vi "Spartan HTTP Load Global Server Configuration.vi"(8 "error in (no error)":errorcluster, 11 "lvhttp.conf":path=path "") -> (0 "error out":errorcluster)   [LabVIEW 2011]
uses:
  ITK EXT/http/http0.llb/HTTP LVHTTP Global.vi
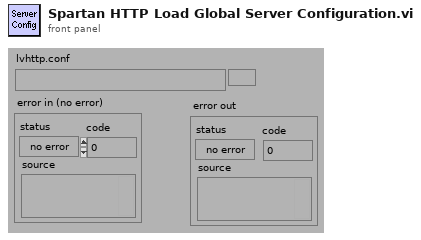
[diagram p1: front panel]
types:
  T1 = typedef "Keyed Array.ctl" = cluster{"keys":string[], "values":string[]}
  T2 = cluster{"[0]":path, "[1]":path, "[2]":path, "[3]":path, "[4]":path, "[5]":path, "[6]":path}
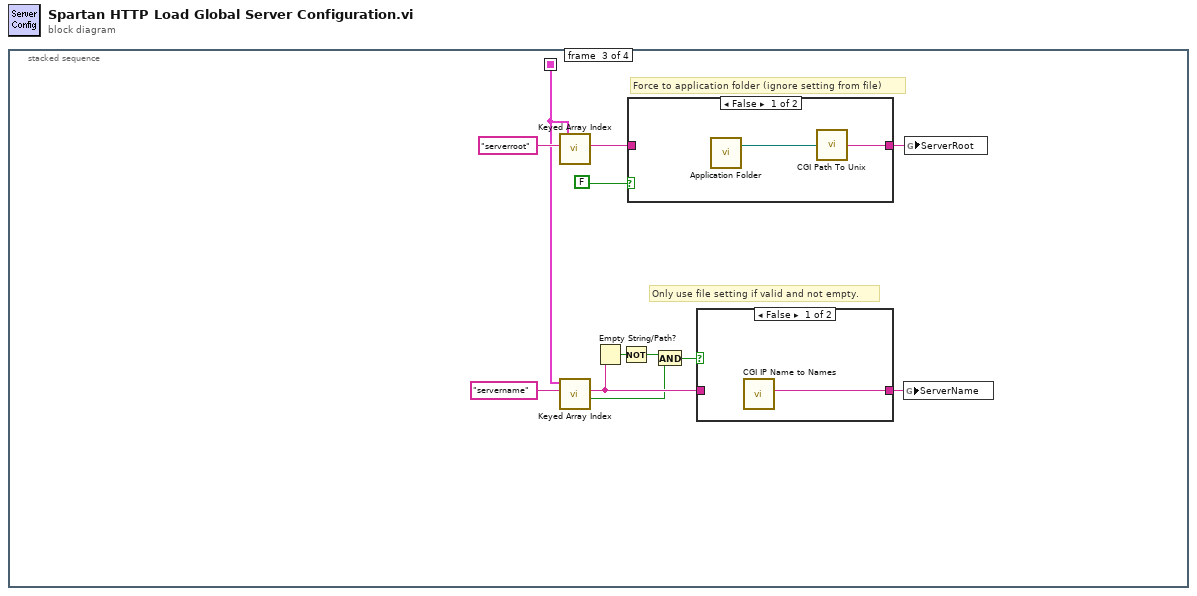
[diagram p0: block diagram]
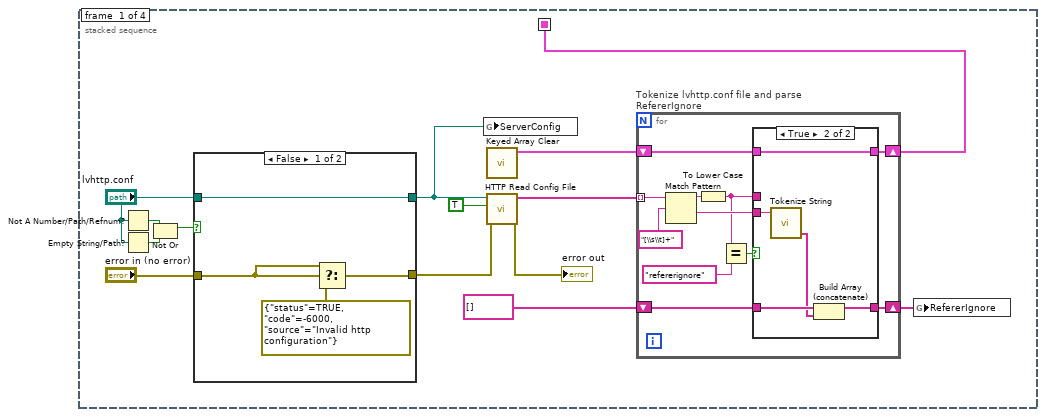
[diagram p2: hidden frame]
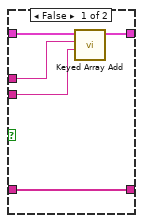
[diagram p4: hidden frame]
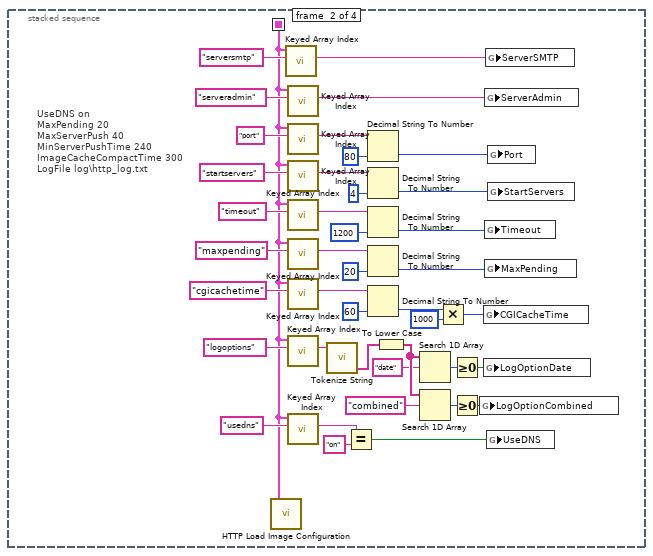
[diagram p5: hidden frame]
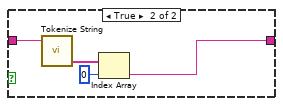
[diagram p7: hidden frame]
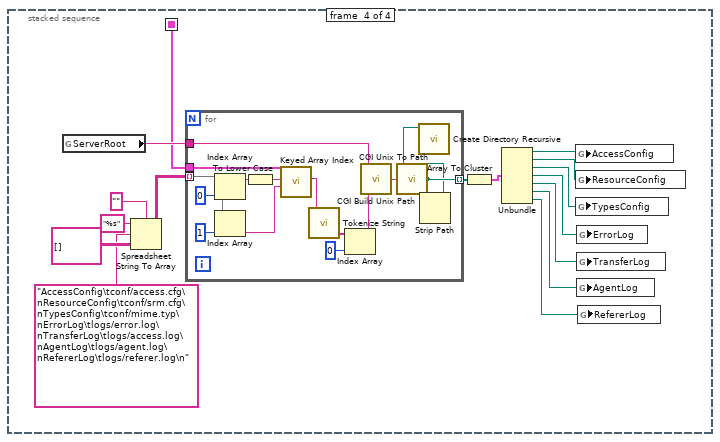
[diagram p8: hidden frame]
diagram:
  n1 = stacked-sequence {
    seq-local: [w9 _ _ _] -> [_ w42 w90 w104]
    frame #0 {
      n2 = Not A Number/Path/Refnum?(number/path/refnum="lvhttp.conf") -> (NaN/Path/Refnum?=w3:bool)
      n3 = Empty String/Path?(string/path="lvhttp.conf") -> (empty?=w4:bool)
      n4 = Not Or(1:w4, 2:w3) -> (0:w1:bool)
      n5 = case shown="False" w1 {
        tunnel: [w15 w20] -> w6
        tunnel: "lvhttp.conf" -> [w15 w20]
        tunnel: "error in (no error)" -> [w18 w19]
        tunnel: [w16 w19] -> w5
        frame False {
          n6 = Select(t=w18, s=w18, f=errorcluster {"status"=TRUE, "code"=-6000, "source"="Invalid http configuration"} ("error out")) -> (s? t:f=w16:errorcluster)
        }
        frame True {
        }
      }
      n7 = global write "HTTP LVHTTP Global.vi" "ServerConfig"(w6) -> ()
      n8 = call "Keyed Array Clear.vi"() -> ("array out"=w10:T1)  [unwired: 1 in, 6 out]
      n9 = call "HTTP Read Config File.vi"("error in (no error)"=w5, "skip blank lines (F)"=TRUE, "config file path"=w6) -> ("error out"=→"error out":errorcluster, "lines"=w13:string[])  [unwired: 7 out]
      n10 = for "Tokenize lvhttp.conf file and parse RefererIgnore" {
        shift-right: [w28] -> w9
        shift-left: w10 -> [w29]
        tunnel: w13 -> [w25] mode=indexing
        shift-right: [w26] -> w11
        shift-left: string[] [] -> [w27]
        n11 = Match Pattern(string=w25, regular expression="[\\s\\t]+") -> (before substring=w24:string, after substring=w23:string)  [unwired: 3 out]
        n12 = To Lower Case(string=w24) -> (all lower case string=w21:string)
        n13 = Equal?(x=w21, y="refererignore") -> (x = y?=w30:bool)
        n14 = case shown="True" w30 {
          tunnel: w29 -> [w36 w41]
          tunnel: w21 -> [w35 _]
          tunnel: [w33 w41] -> w28
          tunnel: w27 -> [w34 w40]
          tunnel: [w34 w39] -> w26
          tunnel: w23 -> [w32 w38]
          frame False {
            n15 = call "Keyed Array Add.vi"("value"=w32, "key"=w35, "array in"=w36) -> ("array out"=w33:T1)  [unwired: 1 in, 3 out]
          }
          frame True {
            n16 = call "Tokenize String.vi"("input string"=w38) -> ("token array"=w37:string[])  [unwired: 1 in, 3 out]
            n17 = Build Array (concatenate)(w40, w37) -> (w39:string[])
          }
        }
      }
      n18 = global write "HTTP LVHTTP Global.vi" "RefererIgnore"(w11) -> ()
    }
    frame #1 {
      # "UseDNS\ton\nMaxPending\t20\nMaxServerPush\t40\nMinServerPushTime 240\nImageCacheCompactTime\t300\nLogFile\tlog\\http_log.txt"
      n19 = call "HTTP Load Image Configuration.vi"("array in"=w42) -> ()  [unwired: 7 out]
      n20 = call "Keyed Array Index.vi"("key"="serversmtp", "array in"=w42) -> ("value"=w44:string)  [unwired: 2 in, 3 out]
      n21 = call "Keyed Array Index.vi"("key"="serveradmin", "array in"=w42) -> ("value"=w73:string)  [unwired: 2 in, 3 out]
      n22 = call "Keyed Array Index.vi"("key"="port", "array in"=w42) -> ("value"=w78:string)  [unwired: 2 in, 3 out]
      n23 = call "Keyed Array Index.vi"("key"="startservers", "array in"=w42) -> ("value"=w76:string)  [unwired: 2 in, 3 out]
      n24 = call "Keyed Array Index.vi"("key"="timeout", "array in"=w42) -> ("value"=w77:string)  [unwired: 2 in, 3 out]
      n25 = call "Keyed Array Index.vi"("key"="maxpending", "array in"=w42) -> ("value"=w67:string)  [unwired: 2 in, 3 out]
      n26 = call "Keyed Array Index.vi"("key"="cgicachetime", "array in"=w42) -> ("value"=w50:string)  [unwired: 2 in, 3 out]
      n27 = call "Keyed Array Index.vi"("key"="logoptions", "array in"=w42) -> ("value"=w60:string)  [unwired: 2 in, 3 out]
      n28 = call "Keyed Array Index.vi"("key"="usedns", "array in"=w42) -> ("value"=w64:string)  [unwired: 2 in, 3 out]
      n29 = call "Tokenize String.vi"("input string"=w60) -> ("token array"=w59:string[])  [unwired: 1 in, 3 out]
      n30 = Equal?(x=w64, y="on") -> (x = y?=w62:bool)
      n31 = Decimal String To Number(string=w78, default (0L)=u16 80) -> (number=w70:u16)  [unwired: 2 out]
      n32 = Decimal String To Number(string=w76, default (0L)=4) -> (number=w71:i32)  [unwired: 2 out]
      n33 = Decimal String To Number(string=w77, default (0L)=1200) -> (number=w72:i32)  [unwired: 2 out]
      n34 = Decimal String To Number(string=w67, default (0L)=20) -> (number=w69:i32)  [unwired: 2 out]
      n35 = Decimal String To Number(string=w50, default (0L)=60) -> (number=w48:i32)  [unwired: 2 out]
      n36 = To Lower Case(string=w59) -> (all lower case string=w58:string[])
      n37 = Search 1D Array(1D array=w58, element="date") -> (index of element=w55:i32)  [unwired: 1 out]
      n38 = Search 1D Array(1D array=w58, element="combined") -> (index of element=w52:i32)  [unwired: 1 out]
      n39 = Multiply(x=w48, y=1000) -> (x*y=w47:i32)
      n40 = Greater Or Equal To 0?(x=w55) -> (x >= 0?=w54:bool)
      n41 = Greater Or Equal To 0?(x=w52) -> (x >= 0?=w53:bool)
      n42 = global write "HTTP LVHTTP Global.vi" "LogOptionCombined"(w53) -> ()
      n43 = global write "HTTP LVHTTP Global.vi" "CGICacheTime"(w47) -> ()
      n44 = global write "HTTP LVHTTP Global.vi" "LogOptionDate"(w54) -> ()
      n45 = global write "HTTP LVHTTP Global.vi" "ServerAdmin"(w73) -> ()
      n46 = global write "HTTP LVHTTP Global.vi" "Timeout"(w72) -> ()
      n47 = global write "HTTP LVHTTP Global.vi" "MaxPending"(w69) -> ()
      n48 = global write "HTTP LVHTTP Global.vi" "ServerSMTP"(w44) -> ()
      n49 = global write "HTTP LVHTTP Global.vi" "UseDNS"(w62) -> ()
      n50 = global write "HTTP LVHTTP Global.vi" "Port"(w70) -> ()
      n51 = global write "HTTP LVHTTP Global.vi" "StartServers"(w71) -> ()
    }
    frame #2 {
      # "Only use file setting if valid and not empty."
      # "Force to application folder (ignore setting from file)"
      n52 = call "Keyed Array Index.vi"("key"="serverroot", "array in"=w90) -> ("value"=w93:string)  [unwired: 2 in, 3 out]
      n53 = call "Keyed Array Index.vi"("key"="servername", "array in"=w90) -> ("valid key"=w85:bool, "value"=w87:string)  [unwired: 2 in, 2 out]
      n54 = Empty String/Path?(string/path=w87) -> (empty?=w86:bool)
      n55 = Not(x=w86) -> (.not. x?=w84:bool)
      n56 = case shown="False" FALSE {
        tunnel: w93 -> [_ w102]
        tunnel: [w98 w99] -> w92
        frame False {
          n57 = call "Application Folder.vi"() -> ("Application Folder"=w97:path)  [unwired: 3 in]
          n58 = call "CGI Path To Unix.vi"("platform path"=w97) -> ("unix path"=w98:string)  [unwired: 1 in]
        }
        frame True {
          n59 = call "Tokenize String.vi"("input string"=w102) -> ("token array"=w101:string[])  [unwired: 1 in, 3 out]
          n60 = Index Array(array=w101, index=0) -> (element=w99:string)
        }
      }
      n61 = And(x=w84, y=w85) -> (x .and. y?=w83:bool)
      n62 = case shown="False" w83 {
        tunnel: w87 -> [_ w96]
        tunnel: [w95 w96] -> w89
        frame False {
          n63 = call "CGI IP Name to Names.vi"() -> ("domain name"=w95:string)  [unwired: 2 in, 5 out]
        }
        frame True {
        }
      }
      n64 = global write "HTTP LVHTTP Global.vi" "ServerName"(w89) -> ()
      n65 = global write "HTTP LVHTTP Global.vi" "ServerRoot"(w92) -> ()
    }
    frame #3 {
      n66 = global read "HTTP LVHTTP Global.vi" "ServerRoot"() -> (w113:string)
      n67 = Spreadsheet String To Array(delimiter (Tab)="", format string="%s", spreadsheet string="AccessConfig\tconf/access.cfg\nResourceConfig\tconf/srm.cfg\nTypesConfig\tconf/mime.typ\nErrorLog\tlogs/error.log\nTransferLog\tlogs/access.log\nAgentLog\tlogs/agent.log\nRefererLog\tlogs/referer.log\n", array type (2D Dbl)=string[][] []) -> (array=w114:string[][])
      n68 = for {
        tunnel: w104 -> [w133]
        tunnel: w114 -> [w130] mode=indexing
        tunnel: w113 -> [w127]
        tunnel: [w120] -> w112 mode=indexing
        n69 = Index Array(array=w130, index=0) -> (element=w129:string)
        n70 = Index Array(array=w130, index=1) -> (element=w128:string)
        n71 = To Lower Case(string=w129) -> (all lower case string=w125:string)
        n72 = call "Keyed Array Index.vi"("default value"=w128, "key"=w125, "array in"=w133) -> ("value"=w124:string)  [unwired: 1 in, 3 out]
        n73 = call "Tokenize String.vi"("input string"=w124) -> ("token array"=w123:string[])  [unwired: 1 in, 3 out]
        n74 = Index Array(array=w123, index=0) -> (element=w121:string)
        n75 = call "CGI Build Unix Path.vi"("absolute or relative path"=w121, "base path"=w127) -> ("new path"=w126:string)
        n76 = call "CGI Unix To Path.vi"("unix path"=w126) -> ("platform path"=w120:path)  [unwired: 1 out]
        n77 = Strip Path(path=w120) -> (stripped path=w119:path)  [unwired: 1 out]
        n78 = call <vilib>:"Create Directory Recursive.vi"("directory"=w119) -> ()  [unwired: 2 in, 5 out]
      }
      n79 = Array To Cluster(array=w112) -> (cluster=w111:T2)
      n80 = Unbundle(w111) -> ("[0]"=w110:path, "[1]"=w103:path, "[2]"=w109:path, "[3]"=w108:path, "[4]"=w107:path, "[5]"=w106:path, "[6]"=w105:path)
      n81 = global write "HTTP LVHTTP Global.vi" "AccessConfig"(w110) -> ()
      n82 = global write "HTTP LVHTTP Global.vi" "ResourceConfig"(w103) -> ()
      n83 = global write "HTTP LVHTTP Global.vi" "TypesConfig"(w109) -> ()
      n84 = global write "HTTP LVHTTP Global.vi" "ErrorLog"(w108) -> ()
      n85 = global write "HTTP LVHTTP Global.vi" "TransferLog"(w107) -> ()
      n86 = global write "HTTP LVHTTP Global.vi" "AgentLog"(w106) -> ()
      n87 = global write "HTTP LVHTTP Global.vi" "RefererLog"(w105) -> ()
    }
  }
